vi "pathPlanner.vi"(8 "Parameters.lvclass":refnum<class "Parameters.lvclass">, 9 "Volta ao redor\nda área?":bool, 10 "Line?":bool, 11 "IA State Output in":T1) -> (3 "IA State Output out":T1)   [LabVIEW 2020]
uses:
  Vision_class/Old vision/SSL Detection Frame Simple Estimator Cameras VelCmd Folder/Core/AI Input.ctl
  Vision_class/Old vision/Controls/AI Robot.ctl
  Vision_class/Old vision/Controls/Functions Enum.ctl
  Vision_class/Old vision/Controls/AttackerStates.ctl
  Vision_class/Old vision/Controls/PathDests.ctl
  Vision_class/Old vision/Controls/PathDest.ctl
  Navigation/VSSNavigation/VSSAttackerStates.ctl
  Vision_class/Old vision/SSL Detection Frame Simple Estimator Cameras VelCmd Folder/Core/AI Ball.ctl
  Vision_class/Old vision/SSL Detection Frame Simple Estimator Cameras VelCmd Folder/Core/Field Size.ctl
  Vision_class/Old vision/SSL Detection Frame Simple Estimator Cameras VelCmd Folder/Core/AI Judge.ctl
  Communication_class/Paths/MessageAI_State Folder/Intel/Command Enum.ctl
  Vision_class/Old vision/SSL Detection Frame Simple Estimator Cameras VelCmd Folder/Util/Events/Events.ctl
  Parameters_class/Parameters.lvclass
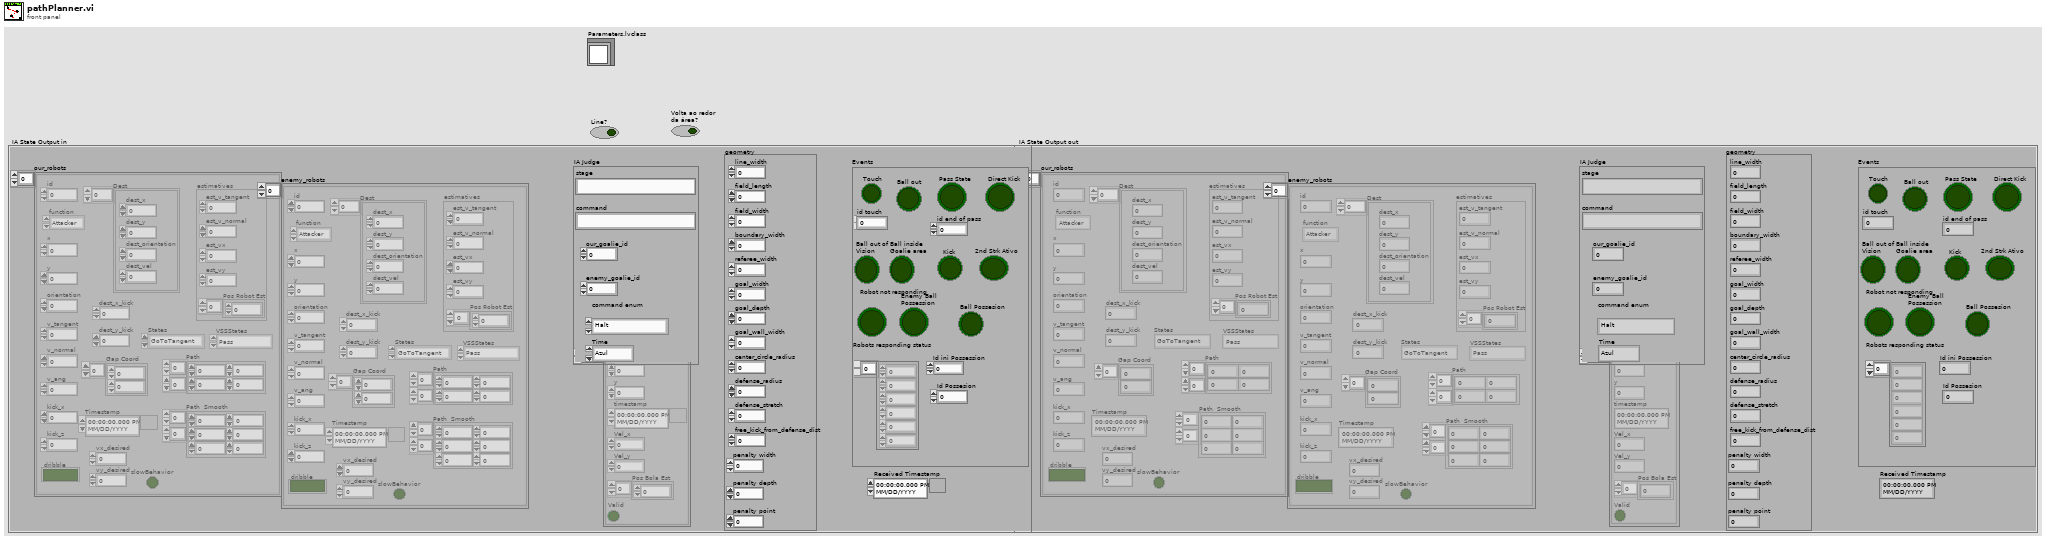
[diagram p1: front panel]
types:
  T1 = typedef "AI Input.ctl" = cluster{"our_robots":T2[], "enemy_robots":T2[], "balls":T8[], "geometry":T9, "IA Judge":T10, "Received Timestamp":timestamp, "Events":T12}
  T2 = typedef "AI Robot.ctl" = cluster{"id":u32, "function":T3, "x":dbl, "y":dbl, "orientation":dbl, "v_tangent":dbl, "v_normal":dbl, "v_ang":dbl, "kick_x":dbl, "kick_z":dbl, "dribble":bool, "Timestamp":timestamp, "estimatives":cluster{"est_v_tangent":dbl, "est_v_normal":dbl, "est_vx":dbl, "est_vy":dbl, "Pos Robot Est":dbl[]}, "dest_x_kick":dbl, "dest_y_kick":dbl, "Gap Coord":dbl[], "States":T4, "Path ":dbl[][], "Path  Smooth":dbl[][], "Dest":T5, "vx_desired":dbl, "vy_desired":dbl, "slowBehavior":bool, "VSSStates":T7}
  T3 = typedef "Functions Enum.ctl" = enum16{"2nd Striker", "Attacker", "Goalie", "Defender", "Striker", "Goto 0", "Dummy", "Kicker", "ZigZag 0", "ZigZag 1", "ZigZag 2", "ZigZag 3", "ZigZag 4", "ZigZag 5", "ZigZag 6", "ZigZag 7", "ZigZag 8", ""}
  T4 = typedef "AttackerStates.ctl" = enum16{"Pass", "GoToTangent", "BallGetting", "GoToKick", ""}
  T5 = typedef "PathDests.ctl" = T6[]
  T6 = typedef "PathDest.ctl" = cluster{"dest_x":dbl, "dest_y":dbl, "dest_orientation":dbl, "dest_vel":dbl}
  T7 = typedef "VSSAttackerStates.ctl" = enum16{"Pass", "GoToTangent", "BallGetting", "GoToKick", "Rotate anti-clockwise", "Rotate Clockwise", ""}
  T8 = typedef "AI Ball.ctl" = cluster{"x":dbl, "y":dbl, "timestamp":timestamp, "Vel_x":dbl, "Vel_y":dbl, "Pos Bola Est":dbl[], "Valid":bool}
  T9 = typedef "Field Size.ctl" = cluster{"line_width":u32, "field_length":u32, "field_width":u32, "boundary_width":u32, "referee_width":u32, "goal_width":u32, "goal_depth":u32, "goal_wall_width":u32, "center_circle_radius":u32, "defense_radius":u32, "defense_stretch":u32, "free_kick_from_defense_dist":u32, "penalty width":dbl, "penalty depth":dbl, "penalty point":dbl}
  T10 = typedef "AI Judge.ctl" = cluster{"stage":string, "command":string, "our_goalie_id":dbl, "enemy_goalie_id":dbl, "command enum":T11, "Time":enum16{"Azul", "Amarelo"}}
  T11 = typedef "Command Enum.ctl" = enum16{"Halt", "Stop", "Force Start", "PKA Normal Start", "Prepare Kickoff Ally", "PKE Normal Start", "Prepare Kickoff Enemy", "Prepare Penalty Ally", "PPA Normal Start", "Prepare Penalty Enemy", "PPE Normal Start", "Direct Free Enemy", "Direct Free Ally", "Indirect Free Enemy", "Indirect Free Ally", "Timeout Enemy", "Timeout Ally", "Goal Enemy", "Goal Ally", "Ball Placement Enemy", "Ball Placement Ally", "Normal Half Time", "Extra Time Break", "Extra Half Time", "None", "Post Game"}
  T12 = typedef "Events.ctl" = cluster{"Touch":bool, "Ball out":bool, "id touch":dbl, "Ball out of \nVision":bool, "Ball inside \nGoalie area":bool, "Robot not responding":bool, "Robots responding status":dbl[], "Enemy Ball \nPossession":bool, "Pass State":bool, "id end of pass":dbl, "Kick":bool, "Id ini Possession":dbl, "Ball Possesion":bool, "Id Possesion":dbl, "Direct Kick":bool, "2nd Strk Ativo":bool}
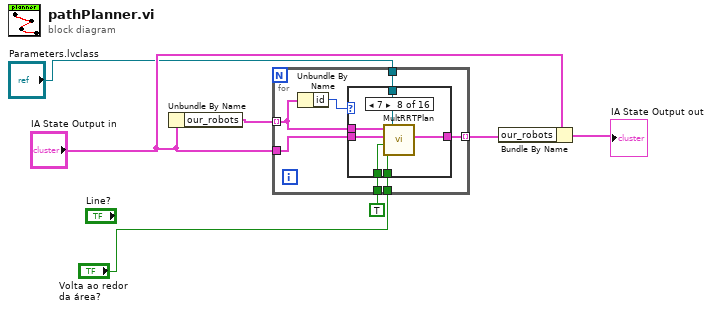
[diagram p0: block diagram]
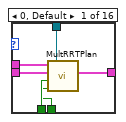
[diagram p2: hidden frame]
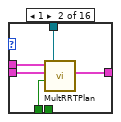
[diagram p3: hidden frame]
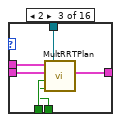
[diagram p4: hidden frame]
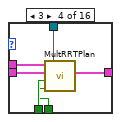
[diagram p5: hidden frame]
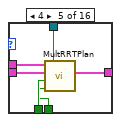
[diagram p6: hidden frame]
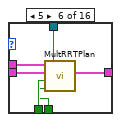
[diagram p7: hidden frame]
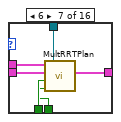
[diagram p8: hidden frame]
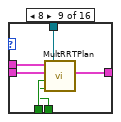
[diagram p9: hidden frame]
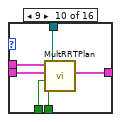
[diagram p10: hidden frame]
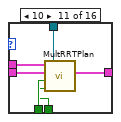
[diagram p11: hidden frame]
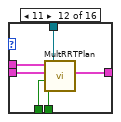
[diagram p12: hidden frame]
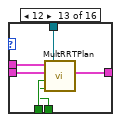
[diagram p13: hidden frame]
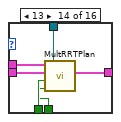
[diagram p14: hidden frame]
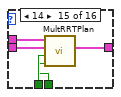
[diagram p15: hidden frame]
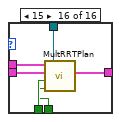
[diagram p16: hidden frame]
diagram:
  n1 = Unbundle By Name("IA State Output in") -> ("our_robots"=w4:T2[])
  n2 = for {
    tunnel: "IA State Output in" -> [w14]
    tunnel: w4 -> [w12] mode=indexing
    tunnel: [w13] -> w5 mode=indexing
    tunnel: TRUE ("Line?") -> [w10]
    tunnel: "Volta ao redor\nda área?" -> [w9]
    tunnel: "Parameters.lvclass" -> [w8]
    n3 = Unbundle By Name(w12) -> ("id"=w11:u32)
    n4 = case shown="7" w11 {
      tunnel: w14 -> [w20 w25 w31 w37 w43 w49 w55 w61 w67 w73 w79 w85 w91 w97 w102 w108]
      tunnel: [w18 w23 w29 w35 w41 w47 w53 w59 w65 w71 w77 w83 w89 w95 w100 w106] -> w13
      tunnel: w12 -> [w19 w24 w30 w36 w42 w48 w54 w60 w66 w72 w78 w84 w90 w96 w101 w107]
      tunnel: w10 -> [w17 w22 w28 w34 w40 w46 w52 w58 w64 w70 w76 w82 w88 w94 w99 w105]
      tunnel: w9 -> [w16 _ w27 w33 w39 w45 w51 w57 w63 w69 w75 w81 w87 w93 w98 w104]
      tunnel: w8 -> [w15 w21 w26 w32 w38 w44 w50 w56 w62 w68 w74 w80 w86 w92 _ w103]
      frame 0, Default {
        n5 = call "MultRRTPlan.vi"("Parameters.lvclass"=w15, "Volta ao redor\nda área?"=w16, "Line?"=w17, "IA State"=w20, "Robot"=w19) -> ("Robot Out"=w18:T2)  [unwired: 6 in]
      }
      frame 1 {
        n6 = call "MultRRTPlan.vi"("Parameters.lvclass"=w21, "Line?"=w22, "IA State"=w25, "Robot"=w24) -> ("Robot Out"=w23:T2)  [unwired: 7 in]
      }
      frame 2 {
        n7 = call "MultRRTPlan.vi"("Parameters.lvclass"=w26, "Volta ao redor\nda área?"=w27, "Line?"=w28, "IA State"=w31, "Robot"=w30) -> ("Robot Out"=w29:T2)  [unwired: 6 in]
      }
      frame 3 {
        n8 = call "MultRRTPlan.vi"("Parameters.lvclass"=w32, "Volta ao redor\nda área?"=w33, "Line?"=w34, "IA State"=w37, "Robot"=w36) -> ("Robot Out"=w35:T2)  [unwired: 6 in]
      }
      frame 4 {
        n9 = call "MultRRTPlan.vi"("Parameters.lvclass"=w38, "Volta ao redor\nda área?"=w39, "Line?"=w40, "IA State"=w43, "Robot"=w42) -> ("Robot Out"=w41:T2)  [unwired: 6 in]
      }
      frame 5 {
        n10 = call "MultRRTPlan.vi"("Parameters.lvclass"=w44, "Volta ao redor\nda área?"=w45, "Line?"=w46, "IA State"=w49, "Robot"=w48) -> ("Robot Out"=w47:T2)  [unwired: 6 in]
      }
      frame 6 {
        n11 = call "MultRRTPlan.vi"("Parameters.lvclass"=w50, "Volta ao redor\nda área?"=w51, "Line?"=w52, "IA State"=w55, "Robot"=w54) -> ("Robot Out"=w53:T2)  [unwired: 6 in]
      }
      frame 7 {
        n12 = call "MultRRTPlan.vi"("Parameters.lvclass"=w56, "Volta ao redor\nda área?"=w57, "Line?"=w58, "IA State"=w61, "Robot"=w60) -> ("Robot Out"=w59:T2)  [unwired: 6 in]
      }
      frame 8 {
        n13 = call "MultRRTPlan.vi"("Parameters.lvclass"=w62, "Volta ao redor\nda área?"=w63, "Line?"=w64, "IA State"=w67, "Robot"=w66) -> ("Robot Out"=w65:T2)  [unwired: 6 in]
      }
      frame 9 {
        n14 = call "MultRRTPlan.vi"("Parameters.lvclass"=w68, "Volta ao redor\nda área?"=w69, "Line?"=w70, "IA State"=w73, "Robot"=w72) -> ("Robot Out"=w71:T2)  [unwired: 6 in]
      }
      frame 10 {
        n15 = call "MultRRTPlan.vi"("Parameters.lvclass"=w74, "Volta ao redor\nda área?"=w75, "Line?"=w76, "IA State"=w79, "Robot"=w78) -> ("Robot Out"=w77:T2)  [unwired: 6 in]
      }
      frame 11 {
        n16 = call "MultRRTPlan.vi"("Parameters.lvclass"=w80, "Volta ao redor\nda área?"=w81, "Line?"=w82, "IA State"=w85, "Robot"=w84) -> ("Robot Out"=w83:T2)  [unwired: 6 in]
      }
      frame 12 {
        n17 = call "MultRRTPlan.vi"("Parameters.lvclass"=w86, "Volta ao redor\nda área?"=w87, "Line?"=w88, "IA State"=w91, "Robot"=w90) -> ("Robot Out"=w89:T2)  [unwired: 6 in]
      }
      frame 13 {
        n18 = call "MultRRTPlan.vi"("Parameters.lvclass"=w92, "Volta ao redor\nda área?"=w93, "Line?"=w94, "IA State"=w97, "Robot"=w96) -> ("Robot Out"=w95:T2)  [unwired: 6 in]
      }
      frame 14 {
        n19 = call "MultRRTPlan.vi"("Volta ao redor\nda área?"=w98, "Line?"=w99, "IA State"=w102, "Robot"=w101) -> ("Robot Out"=w100:T2)  [unwired: 7 in]
      }
      frame 15 {
        n20 = call "MultRRTPlan.vi"("Parameters.lvclass"=w103, "Volta ao redor\nda área?"=w104, "Line?"=w105, "IA State"=w108, "Robot"=w107) -> ("Robot Out"=w106:T2)  [unwired: 6 in]
      }
    }
  }
  n21 = Bundle By Name(cluster="IA State Output in", "our_robots"=w5) -> (→"IA State Output out":T1)
